vi "TestServer.vi"() -> ()   [LabVIEW 2019]
panel:
  in  "unsigned byte array 2":u8[](array[numeric])
  in  "unsigned byte array":u8[](array[numeric])
  in  "Numeric":i32=13
  in  "Data In":u8[](array[numeric])
  in  "stop":bool
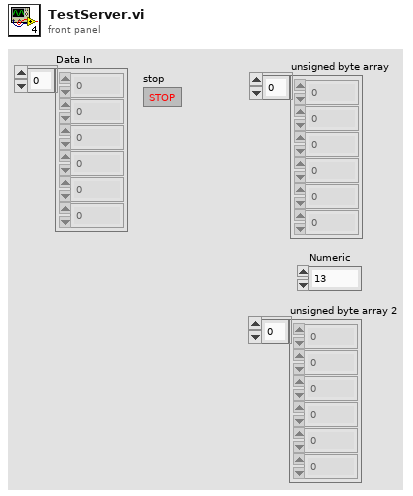
[diagram p1: front panel]
types:
  T1 = enum16{"big-endian, network order", "native, host order", "little-endian"}
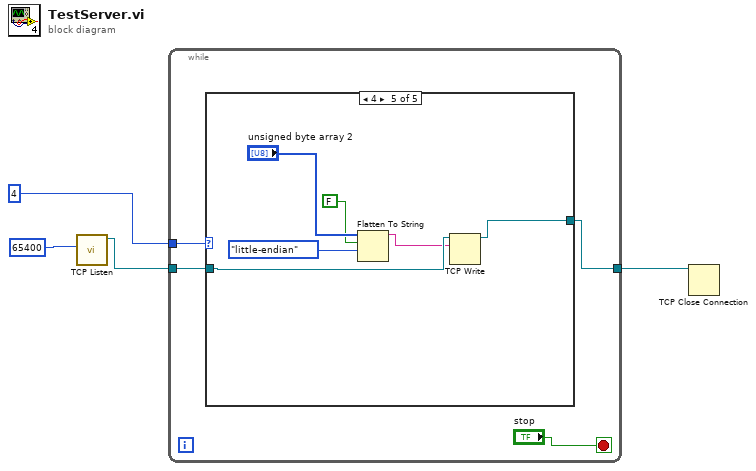
[diagram p0: block diagram]
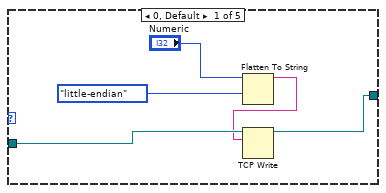
[diagram p2: hidden frame]
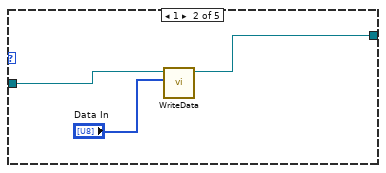
[diagram p3: hidden frame]
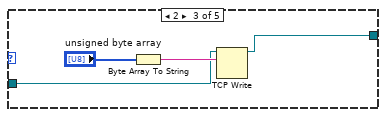
[diagram p4: hidden frame]
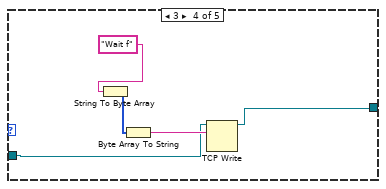
[diagram p5: hidden frame]
diagram:
  n1 = call <vilib>:"TCP Listen.vi"("port"=u32 65400) -> ("connection ID"=w2:refnum<k5>)  [unwired: 6 in, 4 out]
  n2 = while {
    tunnel: 4 -> [w6]
    tunnel: w2 -> [w7]
    tunnel: [w8] -> w4
    stop <- "stop" stop-if-true
    n3 = case shown="4" w6 {
      tunnel: [w12 w16 w17 w24 w30] -> w8
      tunnel: w7 -> [w13 w15 w18 w23 w31]
      frame 0, Default {
        n4 = Flatten To String(anything="Numeric", byte order (0:big-endian, network order)=T1."little-endian") -> (data string=w10:string)  [unwired: 2 in, 2 out]
        n5 = TCP Write(connection ID=w13, data in=w10) -> (connection ID out=w12:refnum<k5>)  [unwired: 2 in, 2 out]
      }
      frame 1 {
        n6 = call "WriteData.vi"("Data In"="Data In", "Connection In"=w15) -> ("Connection Out"=w16:refnum<k5>)  [unwired: 8 in, 1 out]
      }
      frame 2 {
        n7 = Byte Array To String(unsigned byte array="unsigned byte array") -> (string=w20:string)
        n8 = TCP Write(connection ID=w18, data in=w20) -> (connection ID out=w17:refnum<k5>)  [unwired: 2 in, 2 out]
      }
      frame 3 {
        n9 = String To Byte Array(string="Wait f") -> (unsigned byte array=w21:u8[])
        n10 = Byte Array To String(unsigned byte array=w21) -> (string=w25:string)
        n11 = TCP Write(connection ID=w23, data in=w25) -> (connection ID out=w24:refnum<k5>)  [unwired: 2 in, 2 out]
      }
      frame 4 {
        n12 = Flatten To String(anything="unsigned byte array 2", prepend array or string size? (T)=FALSE, byte order (0:big-endian, network order)=T1."little-endian") -> (data string=w28:string)  [unwired: 1 in, 2 out]
        n13 = TCP Write(connection ID=w31, data in=w28) -> (connection ID out=w30:refnum<k5>)  [unwired: 2 in, 2 out]
      }
    }
  }
  n14 = TCP Close Connection(connection ID=w4) -> ()  [unwired: 2 in, 2 out]
